vi "Save Configuration Settings to XML.vi"(8 "error in (no error)":errorcluster caption="错误输入（无错误）", 11 "User Configuration":T1={"Hardware Configuration"={"Physical Channel"="", "Maximum Input"=0.0, "Minimum Input"=0.0, "Sample Rate"=0.0, "Number of Samples"=0}, "Analysis Configuration"={"Statistics"=TRUE}, "New Data Behavior"=enum."Replace"} caption="用户配置") -> (0 "error out":errorcluster caption="错误输出")   [LabVIEW 2013]
doc: "将用户设定的配置数据保存至XML文件。本VI可在多次执行之间保持设置。"
uses:
  controls/User Specified Data.ctl
  controls/HW Configuration.ctl
  controls/Analysis Configuration.ctl
  controls/New Data Behavior.ctl
  <vilib>/Utility/xml.llb/Write to XML File(string).vi
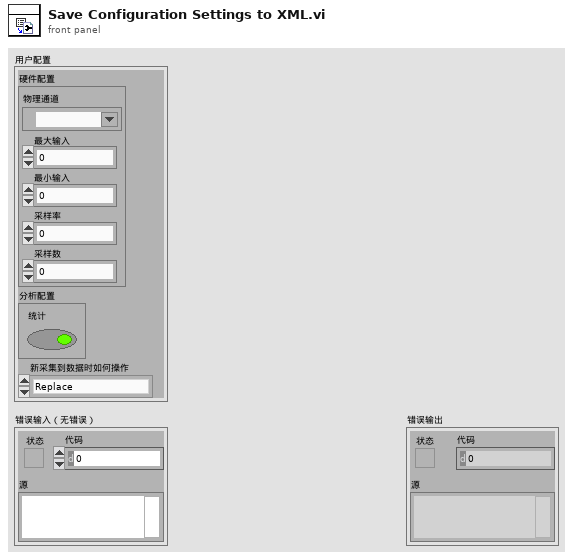
[diagram p1: front panel]
types:
  T1 = typedef "User Specified Data.ctl" = cluster{"Hardware Configuration":T2, "Analysis Configuration":T3, "New Data Behavior":T4}
  T2 = typedef "HW Configuration.ctl" = cluster{"Physical Channel":tag, "Maximum Input":dbl, "Minimum Input":dbl, "Sample Rate":dbl, "Number of Samples":i32}
  T3 = typedef "Analysis Configuration.ctl" = cluster{"Statistics":bool}
  T4 = typedef "New Data Behavior.ctl" = enum16{"Replace", "Overlay", "Append"}
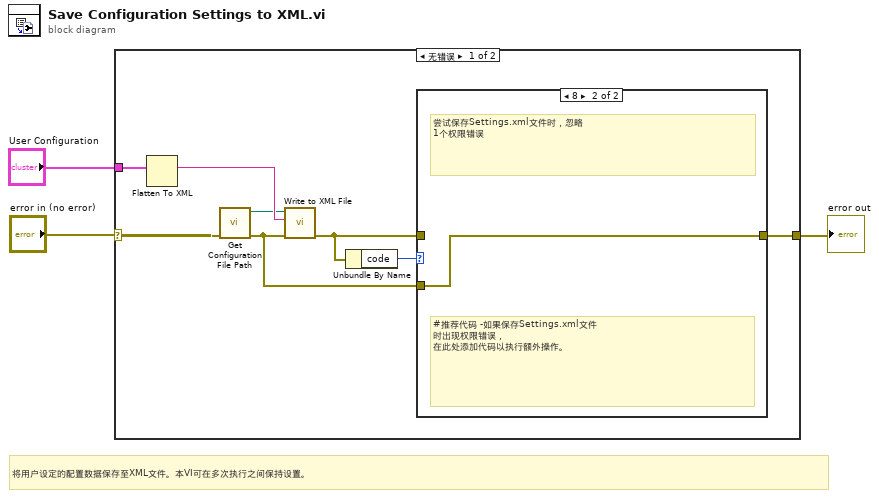
[diagram p0: block diagram]
diagram:
  # "将用户设定的配置数据保存至XML文件。本VI可在多次执行之间保持设置。"
  n1 = case shown="无错误" "error in (no error)" {
    selector: "error in (no error)" -> [w8 w14]
    tunnel: [w5 w14] -> w2
    tunnel: "User Configuration" -> [w11 _]
    frame No Error {
      n2 = Flatten To XML(anything=w11) -> (xml string=w10:string)
      n3 = call "Get Configuration File Path.vi"("error in (no error)"=w8) -> ("error out"=w4:errorcluster, "XML File Path"=w9:path)  [unwired: 9 in]
      n4 = call-poly <vilib>:"Write to XML File.vi"("error in (no error)"=w4, "XML Input"=w10, "XML File Path"=w9) -> ("error out"=w6:errorcluster)  [unwired: 6 in, 2 out]
      n5 = Unbundle By Name(w6) -> ("code"=w7:i32)
      n6 = case shown="8" w7 {
        tunnel: w6 -> [w12 _]
        tunnel: [w12 w13] -> w5
        tunnel: w4 -> [_ w13]
        frame Default {
        }
        frame 8 {
          # "#推荐代码 -如果保存Settings.xml文件\n时出现权限错误，\n在此处添加代码以执行额外操作。"
          # "尝试保存Settings.xml文件时，忽略\n1个权限错误"
        }
      }
    }
    frame Error {
    }
  }
  "error out" <- w2
